vi "Initialize Transfer Groups.vi"(7 "component name":string, 8 "error in (no error)":errorcluster, 10 "Group Configurations":refnum<class "Group Configuration.lvclass">[](array[class]), 11 "UDPlog Transceiver in":refnum<class "UDPlog Transceiver.lvclass">) -> (0 "error out":errorcluster, 3 "UDPlog Transceiver out":refnum<class "UDPlog Transceiver.lvclass">)   [LabVIEW 2023, in "UDPlog.lvlib" / "UDPlog Transceiver.lvclass"]
uses:
  UDPlog Transceiver.lvclass
  UDPlog Transceiver.lvclass/UDPlog Transceiver.ctl
  Typedefs/Transfer Parameters.ctl
  Typedefs/Trasfer Group Parameters.ctl
  <vilib>/AddOns/VeriStand Custom Device Scripting APIs/Data Sharing Framework/DSF Core.lvlibp/Classes/Configuration/Core/Core Configuration.lvclass
  <vilib>/AddOns/VeriStand Custom Device Scripting APIs/Data Sharing Framework/DSF Core.lvlibp/Classes/Configuration/Core/Group/Group Configuration.lvclass
  C:/Program Files/National Instruments/LabVIEW 2023/Vi.Lib/AddOns/VeriStand Custom Device Scripting APIs/Data Sharing Framework/DSF Core.lvlibp/Classes/Configuration/Core/Core Configuration.lvclass
  C:/Program Files/National Instruments/LabVIEW 2023/Vi.Lib/AddOns/VeriStand Custom Device Scripting APIs/Data Sharing Framework/DSF Core.lvlibp/Classes/Configuration/Configuration.lvclass
  C:/Program Files/National Instruments/LabVIEW 2023/Vi.Lib/AddOns/VeriStand Custom Device Scripting APIs/Data Sharing Framework/DSF Core.lvlibp/Classes/Configuration/Core/Group/Group Configuration.lvclass
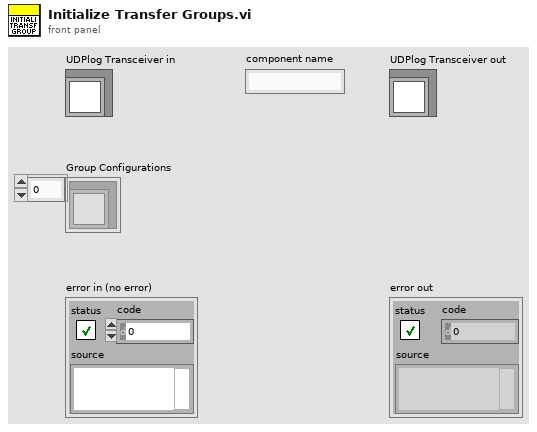
[diagram p1: front panel]
types:
  T1 = typedef "UDPlog.lvlib/UDPlog Transceiver.lvclass/Trasfer Group Parameters.ctl" = cluster{"transfers":T2[], "max size":i32, "timeout":i32}
  T2 = typedef "UDPlog.lvlib/UDPlog Transceiver.lvclass/Transfer Parameters.ctl" = cluster{"group offset":u64, "size":u64, "address":u32, "port":u16}
  T3 = typedef "DSF Core.lvlibp/Group Configuration.lvclass/Core Group Configuration.ctl" = cluster{"name":string, "direction":T4, "cycle timing":T5, "timeout behavior":T6, "enable conversion":bool}
  T4 = typedef "DSF Core.lvlibp/DSF Direction.ctl" = enum8{"Tx", "Rx"}
  T5 = typedef "DSF Core.lvlibp/DSF Timing Info.ctl" = cluster{"priority":u64, "decimation":u64, "offset":u64}
  T6 = typedef "DSF Core.lvlibp/DSF Timeout Behavior.ctl" = enum8{"Increment Late Count", "Throw Error"}
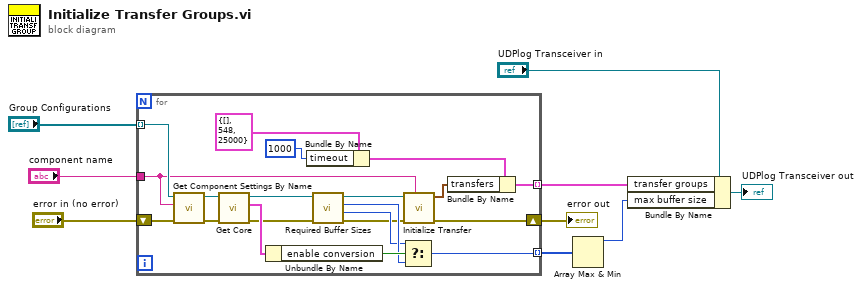
[diagram p0: block diagram]
diagram:
  n1 = for {
    shift-right: [w13] -> w6
    shift-left: "error in (no error)" -> [w25]
    tunnel: "Group Configurations" -> [w26] mode=indexing
    tunnel: [w12] -> w4 mode=indexing
    tunnel: "component name" -> [w15]
    tunnel: [w10] -> w1 mode=indexing
    n2 = call <vilib>:"Get Component Settings By Name.vi"("error in (no error)"=w25, "component name"=w15, "Runtime Configuration in"=w26) -> ("error out"=w23:errorcluster, "Runtime Configuration out"=w24:refnum<class "Group Configuration.lvclass">)  [unwired: 6 in, 1 out]
    n3 = call <vilib>:"Get Core.vi"("error in (no error)"=w23, "Group Configuration in"=w24) -> ("error out"=w20:errorcluster, "core"=w22:T3, "Group Configuration out"=w21:refnum<class "Group Configuration.lvclass">)  [unwired: 7 in]
    n4 = Unbundle By Name(w22) -> ("enable conversion"=w19:bool)
    n5 = Bundle By Name(cluster=T1 {"transfers"=[], "max size"=548, "timeout"=25000} ("transfer group"), "timeout"=1000) -> (w27:T1)
    n6 = call-dynamic "Required Buffer Sizes.vi"("error in (no error)"=w20, "Group Configuration in"=w21) -> ("error out"=w14:errorcluster, "string size"=w17:u64, "engine size"=w18:u64, "Group Configuration out"=w16:refnum<class "Group Configuration.lvclass">)  [unwired: 6 in]
    n7 = Select(t=w17, s=w19, f=w18) -> (s? t:f=w10:u64)
    n8 = call "Initialize Transfer.vi"("component name"=w15, "error in (no error)"=w14, "Group Configuration"=w16) -> ("error out"=w13:errorcluster, "transfer parameters"=w11:T2[])  [unwired: 7 in]
    n9 = Bundle By Name(cluster=w27, "transfers"=w11) -> (w12:T1)
  }
  "error out" <- w6
  n10 = Array Max & Min(array=w1) -> (max value=w3:u64)  [unwired: 3 out]
  n11 = Bundle By Name(cluster="UDPlog Transceiver in", "transfer groups"=w4, "max buffer size"=w3) -> (→"UDPlog Transceiver out":refnum<class "UDPlog Transceiver.lvclass">)
